vi "Funcionamento de bibliotecas.vi"() -> ()   [LabVIEW 2022 SP3]
panel:
  in  "z":string
  in  "y":string
  in  "x":string
  in  "plot path":path=path "C:/Users/chericks/Desktop/Python/LabVIEW/plot.jpeg"
  out "Plot":picture
  out "error out":errorcluster
  out "return value":string
  in  "module path":path=path "C:/Users/chericks/Desktop/Python/LabVIEW/numpy_example.py"
  in  "function name":string="function"
  in  "error in (no error)":errorcluster
  in  "Python version":string="3.6"
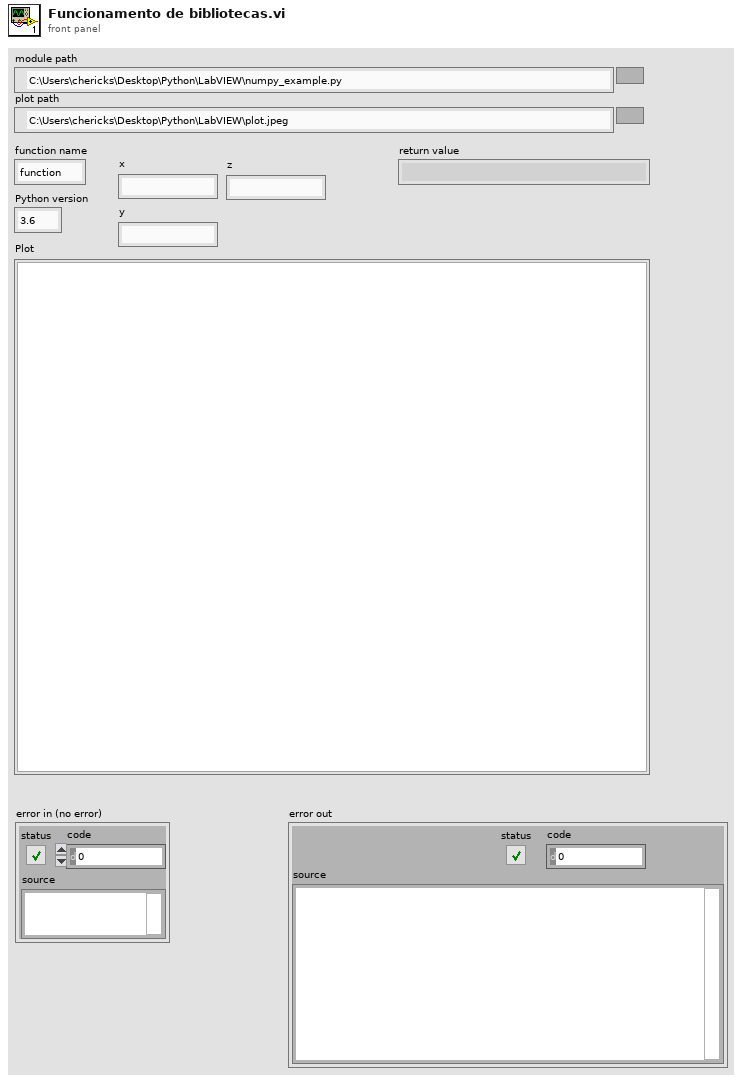
[diagram p1: front panel]
types:
  T1 = typedef "imagedata.ctl" = cluster{"image type":i32, "image depth":i32, "image":u8[], "mask":u8[], "colors":u32[], "Rectangle":cluster{"left":i16, "top":i16, "right":i16, "bottom":i16}}
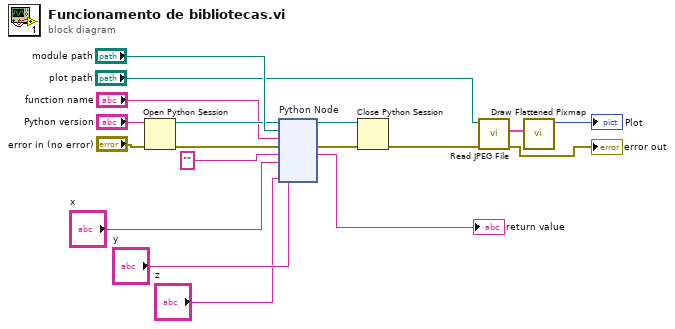
[diagram p0: block diagram]
diagram:
  n1 = Open Python Session(python version="Python version", 3:"error in (no error)") -> (session out=w13:refnum<k35>, error out=w15:errorcluster)  [unwired: 1 in]
  n2 = node "Python Node"(w13, "module path", "function name", w15, "", "x", "y", "z") -> (w12:refnum<k35>, w14:errorcluster, →"return value":string)  [unwired: 3 in, 2 out]
  n3 = Close Python Session(session in=w12, error in=w14) -> (11:w8:errorcluster)
  n4 = call <vilib>:"Read JPEG File.vi"("error in (no error)"=w8, "path to JPEG file"="plot path") -> ("error out"=→"error out":errorcluster, "image data"=w10:T1)  [unwired: 7 in, 1 out]
  n5 = call <vilib>:"Draw Flattened Pixmap.vi"("image data"=w10) -> ("new picture"=→"Plot":picture)  [unwired: 8 in]
